vi "Create Log Page.vi"(7 "Root Path":path, 8 "error in (no error)":errorcluster, 11 "Report In":refnum<class "NI_report.lvclass">) -> (0 "error out":errorcluster, 3 "Report Out":refnum<class "NI_report.lvclass">)   [LabVIEW 2014]
uses:
  <vilib>/Utility/NIReport.llb/NI_report.lvclass
  <vilib>/addons/_office/excel.llb/Excel Easy Table (str).vi
  <vilib>/Utility/NIReport.llb/Append Image to Report (path wrap).vi
  <vilib>/addons/_office/NI_ReportGenerationToolkit.lvlib
  <vilib>/Utility/NIReport.llb/Excel/NI_Excel.lvclass
panel:
  in  "Start Cell":cluster{"row":i32, "column":i32}={"row"=3, "column"=0}
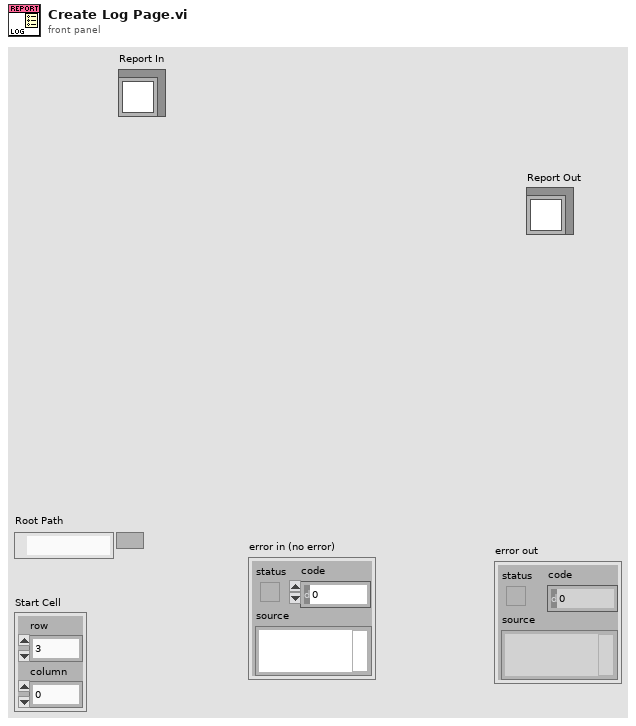
[diagram p1: front panel]
types:
  T1 = cluster{"position (Excel)":cluster{"row":i32, "column":i32}, "name (Excel)":string, "bookmark (Word)":string}
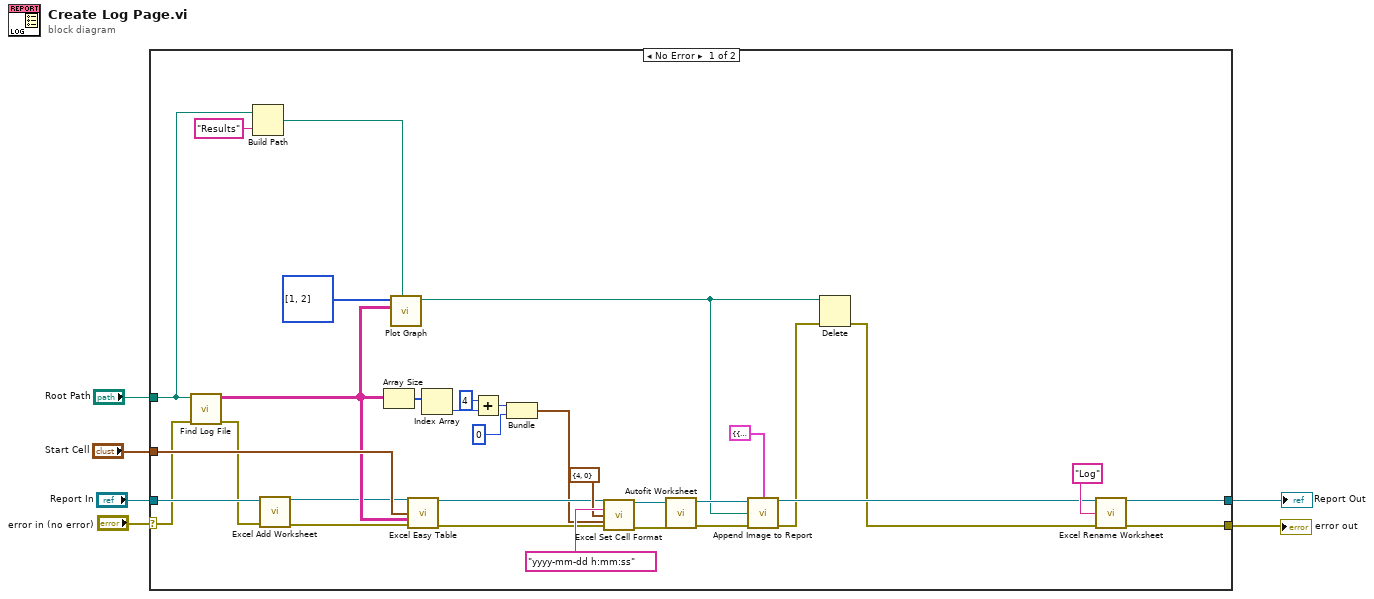
[diagram p0: block diagram]
diagram:
  n1 = case shown="No Error" "error in (no error)" {
    selector: "error in (no error)" -> [w34 w41]
    tunnel: [w37 w41] -> w6
    tunnel: "Report In" -> [w38 w40]
    tunnel: [w36 w40] -> w3
    tunnel: "Start Cell" -> [w39 _]
    tunnel: "Root Path" -> [w20 _]
    frame No Error {
      n2 = call "Find Log File.vi"("error in (no error)"=w34, "Root Path"=w20) -> ("error out"=w33:errorcluster, "Log Data"=w18:string[][])  [unwired: 8 in]
      n3 = Build Path(base path=w20, name or relative path="Results") -> (appended path=w17:path)
      n4 = call <vilib>:"Excel Add Worksheet.vi"("report in"=w38, "error in (no error)"=w33) -> ("report out"=w12:refnum<class "NI_report.lvclass">, "error out"=w11:errorcluster)  [unwired: 12 in]
      n5 = Array Size(array=w18) -> (size(s)=w28:i32[])
      n6 = call "Plot Graph.vi"("path to PNG file"=w17, "Log Data"=w18, "Indexes"=i32[] [1, 2]) -> ("Plot Path"=w10:path)  [unwired: 8 in]
      n7 = call-poly <vilib>:"Excel Easy Table.vi"("report in"=w12, "start (0, 0)"=w39, "text data"=w18, "error in (no error)"=w11) -> ("report out"=w30:refnum<class "NI_report.lvclass">, "error out"=w29:errorcluster)  [unwired: 7 in, 3 out]
      n8 = Index Array(array=w28) -> (element=w27:i32)  [unwired: 1 in]
      n9 = Add(x=4, y=w27) -> (x+y=w22:i32)
      n10 = Bundle(w22, "element"=0) -> (w25:cluster{i32, "element":i32})  [unwired: 1 in]
      n11 = call <vilib>:"Excel Set Cell Format.vi"("report in"=w30, "number format"="yyyy-mm-dd h:mm:ss", "start (-1, -1)"=cluster{"row":i32, "column":i32} {"row"=4, "column"=0}, "end (-1, -1)"=w25, "error in (no error)"=w29) -> ("report out"=w23:refnum<class "NI_report.lvclass">, "error out"=w24:errorcluster)  [unwired: 9 in]
      n12 = call "Autofit Worksheet.vi"("error in (no error)"=w24, "Report In"=w23) -> ("error out"=w16:errorcluster, "Report Out"=w15:refnum<class "NI_report.lvclass">)  [unwired: 8 in]
      n13 = call-poly <vilib>:"Append Image to Report.vi"("report in"=w15, "MS Office parameters"=T1 {"position (Excel)"={"row"=0, "column"=12}, "name (Excel)"="", "bookmark (Word)"=""}, "path or URL of image"=w10, "error in (no error)"=w16) -> ("report out"=w14:refnum<class "NI_report.lvclass">, "error out"=w9:errorcluster)  [unwired: 8 in, 2 out]
      n14 = Delete(path (use dialog)=w10, error in=w9) -> (error out=w8:errorcluster)  [unwired: 3 in, 2 out]
      n15 = call <vilib>:"Excel Rename Worksheet.vi"("report in"=w14, "worksheet name (\"\")"="Log" ("worksheet name (\"\")"), "error in (no error)"=w8) -> ("report out"=w36:refnum<class "NI_report.lvclass">, "error out"=w37:errorcluster)  [unwired: 11 in]
    }
    frame Error {
    }
  }
  "error out" <- w6
  "Report Out" <- w3
